vi "New.vi"(10 "Reseek after # bad polarizations (4)":u32=4, 11 "Number of samples (3)":i32=3) -> (0 "error out":errorcluster, 3 "Automatic Mode out":refnum<class "Automatic Mode.lvclass">)   [LabVIEW 2018, in "Automatic Mode.lvclass"]
uses:
  Automatic Mode.lvclass
  Automatic Mode.lvclass/Automatic Mode.ctl
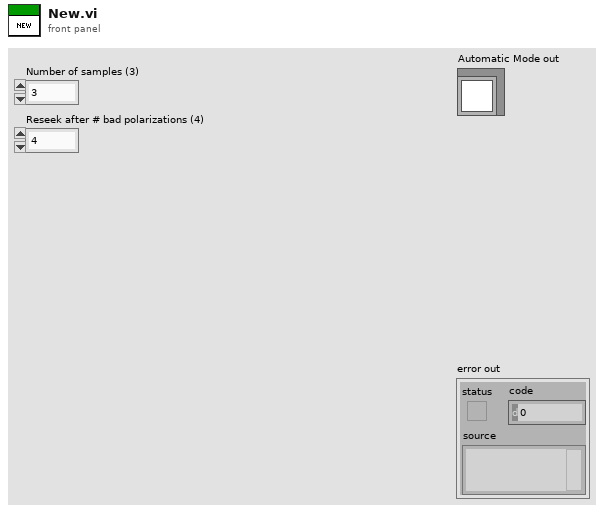
[diagram p1: front panel]
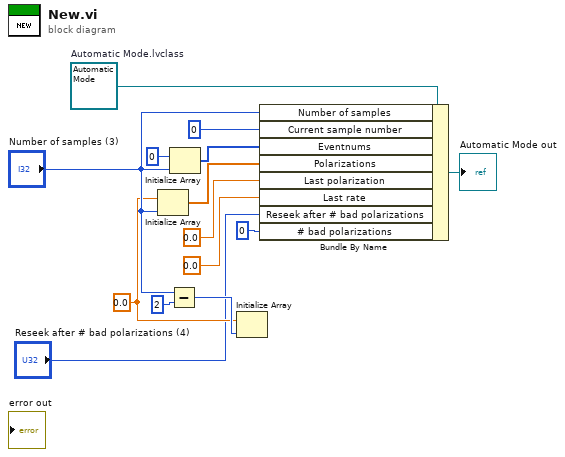
[diagram p0: block diagram]
diagram:
  w9 = 0.0 ("element")
  w14 = refnum<class "Automatic Mode.lvclass"> refnum  # Automatic Mode.lvclass
  n1 = Initialize Array(w9, "Number of samples (3)") -> (w6:dbl[])
  n2 = Subtract(x="Number of samples (3)", y=2) -> (x-y=w12:i32)
  n3 = Initialize Array(i64 0 ("element"), "Number of samples (3)") -> (w7:i64[])
  n4 = Initialize Array(w9, w12) -> ()  [unwired: 1 out]
  n5 = Bundle By Name(cluster=w14, "Number of samples"="Number of samples (3)", "Current sample number"=0, "Eventnums"=w7, "Polarizations"=w6, "Last polarization"=0.0, "Last rate"=0.0, "Reseek after # bad polarizations"="Reseek after # bad polarizations (4)", "# bad polarizations"=u32 0) -> (→"Automatic Mode out":refnum<class "Automatic Mode.lvclass">)
